vi "Agilent 3352X Series Arbitrary Waveform.vi"() -> ()   [LabVIEW 2019]
doc: "This example shows how to create then configure an arbitrary waveform."
uses:
  Instance           2 47Saved   Agilent 3352X Series Arbitrary Waveform .vi
  Instance           1 47Saved   Agilent 3352X Series Arbitrary Waveform .vi
  <instrlib>/Agilent 3352X Series/Agilent 3352X Series.lvlib
panel:
  in  "Offset (0.00 V)":dbl
  in  "Sample Rate (4000 Sa/s)":dbl=4000.0
  in  "Gain (0.1 Vpp)":dbl=0.1
  in  "Arbitrary Waveform Name":string="ARB1"
  in  "VISA resource name":refnum<visa-resource-name>
  # "(c) 2011-2019  National Instruments.  ALL RIGHTS RESERVED."
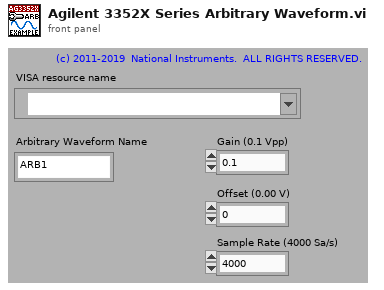
[diagram p1: front panel]
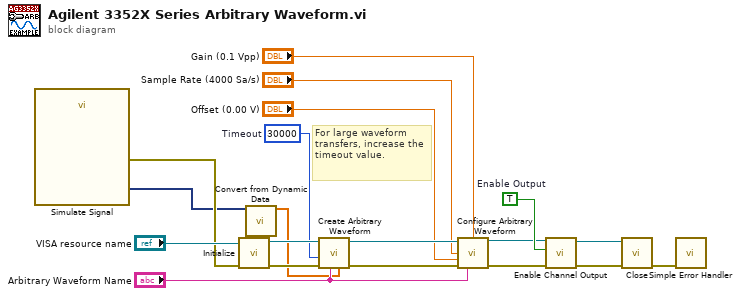
[diagram p0: block diagram]
diagram:
  w12 = TRUE  # Enable Output
  w3 = u32 30000  # Timeout
  # "For large waveform transfers, increase the timeout value."
  n1 = call "Simulate Signal"() -> ("Sine with Uniform Noise"=w2:dynamicdata, "error out"=w18:errorcluster)  [unwired: 8 in, 6 out]
  n2 = call <instrlib>:"Initialize.vi"("error in (no error)"=w18, "VISA resource name"="VISA resource name") -> ("error out"=w14:errorcluster, "VISA resource name out"=w13:refnum<visa-resource-name>)  [unwired: 2 in, 6 out]
  n3 = call "Convert from Dynamic Data"("Dynamic Data Type"=w2) -> ("Array"=w1:dbl[])  [unwired: 3 in]
  n4 = call <instrlib>:"Create Arbitrary Waveform.vi"("Arbitrary Waveform Data"=w1, "Arbitrary Waveform Name (ARB1)"="Arbitrary Waveform Name", "error in (no error)"=w14, "Timeout (10000 ms)"=w3, "VISA resource name"=w13) -> ("error out"=w10:errorcluster, "VISA resource name out"=w11:refnum<visa-resource-name>)  [unwired: 2 in, 3 out]
  n5 = call <instrlib>:"Configure Arbitrary Waveform.vi"("VISA resource name"=w11, "Amplitude (0.1 Vpp)"="Gain (0.1 Vpp)", "Sample Rate (40000 Sa/s)"="Sample Rate (4000 Sa/s)", "Offset (0 V)"="Offset (0.00 V)", "error in (no error)"=w10, "Arbitrary Waveform (ARB1)"="Arbitrary Waveform Name") -> ("VISA resource name out"=w8:refnum<visa-resource-name>, "error out"=w9:errorcluster)  [unwired: 4 in, 4 out]
  n6 = call <instrlib>:"Enable Channel Output.vi"("error in (no error)"=w9, "Enable Output (T: Enable)"=w12, "VISA resource name"=w8) -> ("error out"=w16:errorcluster, "VISA resource name out"=w15:refnum<visa-resource-name>)  [unwired: 2 in, 5 out]
  n7 = call <instrlib>:"Close.vi"("error in (no error)"=w16, "VISA resource name"=w15) -> ("error out"=w17:errorcluster)  [unwired: 9 out]
  n8 = call <vilib>:"Simple Error Handler.vi"("error in (no error)"=w17) -> ()  [unwired: 1 in, 8 out]
